vi "输入框.vi"(1 "提示信息":string) -> (0 "条形码输出":string)   [LabVIEW 2018]
panel:
  in  "字符串":string
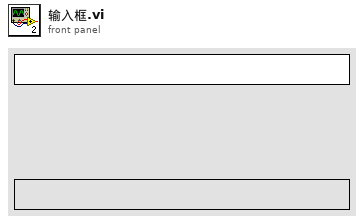
[diagram p1: front panel]
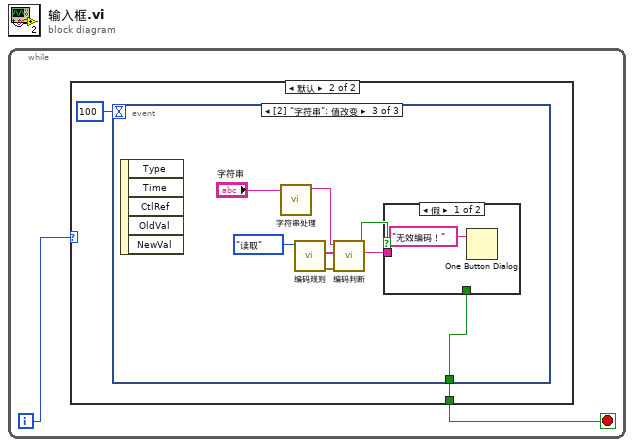
[diagram p0: block diagram]
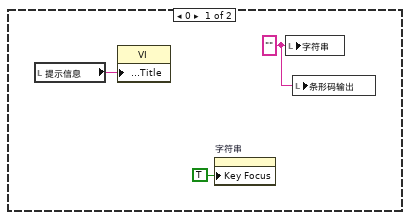
[diagram p2: hidden frame]
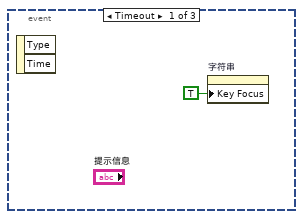
[diagram p3: hidden frame]
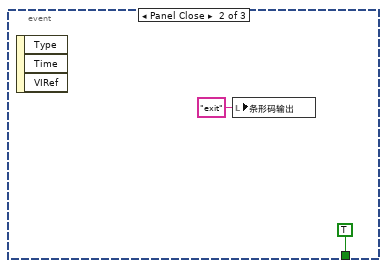
[diagram p4: hidden frame]
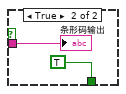
[diagram p5: hidden frame]
diagram:
  n1 = while {
    i -> [w1]
    stop <- w2 stop-if-true
    n2 = case shown="默认" w1 {
      tunnel: [_ w7] -> w2
      frame 0 {
        w5 = "" ("字符串")
        n3 = local read "提示信息"() -> (w4:string)
        n4 = property class="VI"("Front Panel.Title"=w4) -> ()  [unwired: 2 in, 2 out]
        n5 = property on="字符串" class="Str"("Key Focus"=TRUE ("键选中")) -> ()  [unwired: 2 in, 2 out]
        n6 = local write "字符串"(w5) -> ()
        n7 = local write "条形码输出"(w5) -> ()
      }
      frame Default {
        n8 = event shown="[2] \"字符串\": 值改变" {
          selector: _ -> [_ _ _]
          dyn-events: _ -> [_ _ _]
          timeout: 100 -> [_ _ _]
          tunnel: [_ TRUE w13] -> w7
          event Timeout {
            n9 = event-data() -> ()  [unwired: 1 in, 2 out]
            n10 = property on="字符串" class="Str"("Key Focus"=TRUE ("键选中")) -> ()  [unwired: 2 in, 2 out]
          }
          event Panel Close {
            n11 = event-data() -> ()  [unwired: 1 in, 3 out]
            n12 = local write "条形码输出"("exit" ("条形码输出")) -> ()
          }
          event "字符串": Value Change {
            n13 = event-data() -> ()  [unwired: 1 in, 5 out]
            n14 = call "字符串处理.vi"("输入字符串"="字符串") -> ("输出字符串"=w11:string)  [unwired: 10 in]
            n15 = call "编码规则.vi"("功能"=enum16{"读取", "写入"}."读取") -> ("错误输出"=w17:errorcluster, "正则表达式输出（多行）"=w18:string[])  [unwired: 8 in, 1 out]
            n16 = call "编码判断.vi"("错误输入"=w17, "编码规则"=w18, "输入编码"=w11) -> ("输出编码"=w15:string, "有效编码？"=w14:bool)  [unwired: 6 in, 1 out]
            n17 = case shown="假" w14 {
              tunnel: w15 -> [_ w21]
              tunnel: [_ TRUE] -> w13
              frame False {
                n18 = One Button Dialog(message="无效编码！" ("消息")) -> ()  [unwired: 1 in, 1 out]
              }
              frame True {
                "条形码输出" <- w21
              }
            }
          }
        }
      }
    }
  }
